vi "AttrMapToCluster.vi"(8 "error in (no error)":errorcluster, 11 "AttrMap":T1) -> (0 "error out":errorcluster, 3 "Cluster":variant)   [LabVIEW 2019, in "lv-apt-json-file.lvlib"]
uses:
  lv-apt-json-file.lvlib
  Typedef/Def-AttrMap.ctl
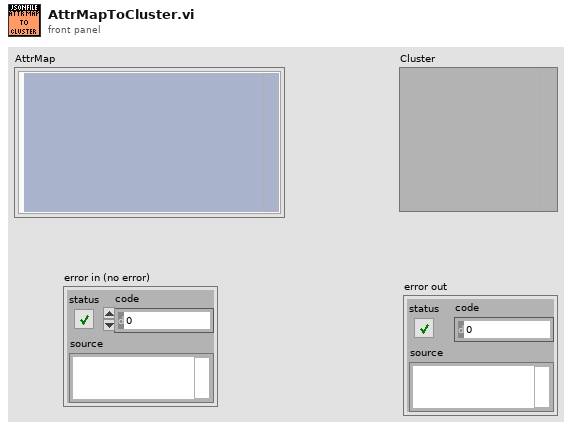
[diagram p1: front panel]
types:
  T1 = typedef "lv-apt-json-file.lvlib/Def-AttrMap.ctl" = cluster{"Map":variant}
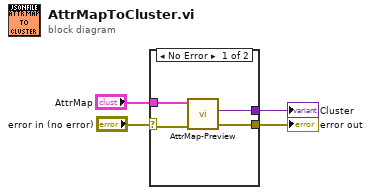
[diagram p0: block diagram]
diagram:
  n1 = case shown="No Error" "error in (no error)" {
    selector: "error in (no error)" -> [w8 w9]
    tunnel: [w5 w9] -> w4
    tunnel: "AttrMap" -> [w7 _]
    tunnel: [w6 _] -> w1
    frame No Error {
      n2 = call "AttrMap-Preview.vi"("error in (no error)"=w8, "AttrMap in"=w7) -> ("error out"=w5:errorcluster, "data"=w6:variant)  [unwired: 7 in, 1 out]
    }
    frame Error {
    }
  }
  "Cluster" <- w1
  "error out" <- w4
